vi "Butterfly Values to Publishable Names.vi"(1 "Butterfly Numbers":dbl[](array[numeric])) -> (0 "Publishable Names":string[](array[string]))   [LabVIEW 2013]
doc: "This VI converts an array of numbers to strings, and appends the \"PI_\" to the rising numbers and \"RL_\" to the falling numbers according to a general butterfly curve."
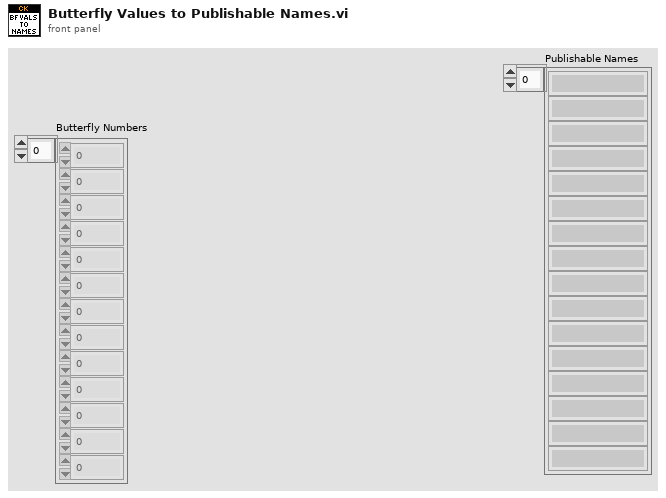
[diagram p1: front panel]
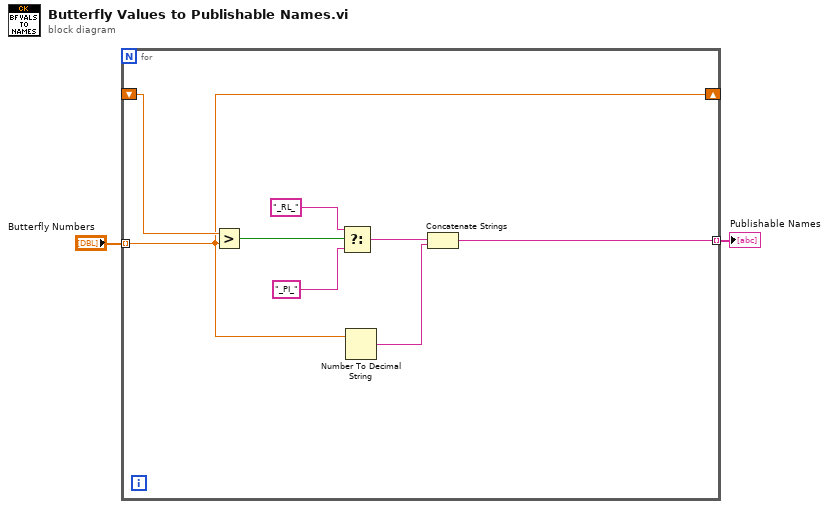
[diagram p0: block diagram]
diagram:
  n1 = for {
    tunnel: "Butterfly Numbers" -> [w6] mode=indexing
    shift-right: [w6] -> _
    shift-left: _ -> [w10]
    tunnel: [w3] -> w1 mode=indexing
    n2 = Greater?(x=w10, y=w6) -> (0:w9:bool)
    n3 = Select(t="_RL_", s=w9, f="_PI_") -> (s? t:f=w5:string)
    n4 = Number To Decimal String(number=w6) -> (decimal integer string=w4:string)  [unwired: 1 in]
    n5 = Concatenate Strings(w5, w4) -> (w3:string)
  }
  "Publishable Names" <- w1
